vi "configuration.set.vi"(8 "error in":errorcluster, 11 "configuration":T1={"Position"=enum."Left", "Note Length"=50.0} {"Note Length" format="%#_13g"}) -> (0 "error out":errorcluster)   [LabVIEW 2020]
uses:
  configuration.ctl
  <vilib>/Utility/config.llb/NI_LVConfig.lvlib
  <userlib>/_OpenG.lib/variantconfig/variantconfig.llb/openg_variant_configuration_file.lvlib
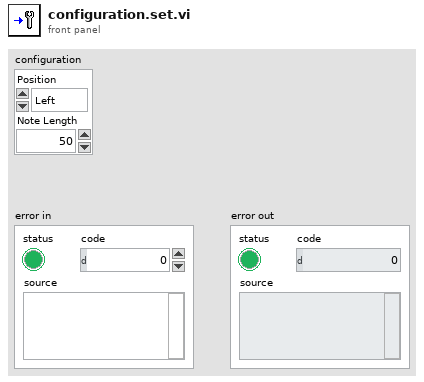
[diagram p1: front panel]
types:
  T1 = typedef "configuration.ctl" = cluster{"Position":enum16{"Top", "Left", "Botom", "Right"}, "Note Length":dbl}
  T2 = typedef "NI_LVConfig.lvlib/Config Data RefNum.ctl" = refnum<k1>
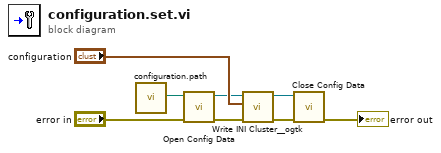
[diagram p0: block diagram]
diagram:
  n1 = call "configuration.path.vi"() -> ("configuration file"=w1:path)  [unwired: 11 in]
  n2 = call <vilib>:"Open Config Data.vi"("error in (no error)"="error in", "configuration file path"=w1) -> ("error out"=w4:errorcluster, "refnum"=w5:T2)  [unwired: 7 in, 1 out]
  n3 = call <userlib>:"Write INI Cluster__ogtk.vi"("error in (no error)"=w4, "INI Fomatted Cluster"="configuration", "refnum"=w5) -> ("error out"=w3:errorcluster, "dup refnum"=w2:T2)  [unwired: 7 in]
  n4 = call <vilib>:"Close Config Data.vi"("error in (no error)"=w3, "refnum"=w2) -> ("error out"=→"error out":errorcluster)  [unwired: 8 in, 1 out]
